vi "Get_All_Sensor_Inputs.vi"(11 "Camera Inputs":T1) -> (3 "Input_Sensors":T2)   [LabVIEW 2012]
uses:
  Inputs_All.ctl
  Flywheel/Sensor_Inputs_FlyWheel.ctl
  tankdrive/Input_Sensors_Drive.ctl
  Conveyor/Sensor_Input_Conveyor.ctl
  Conveyor/Sensor_Input_ConveyorV2.ctl
  Turret/Inputs_Sensors_Turret.ctl
  Inputs_Camera.ctl
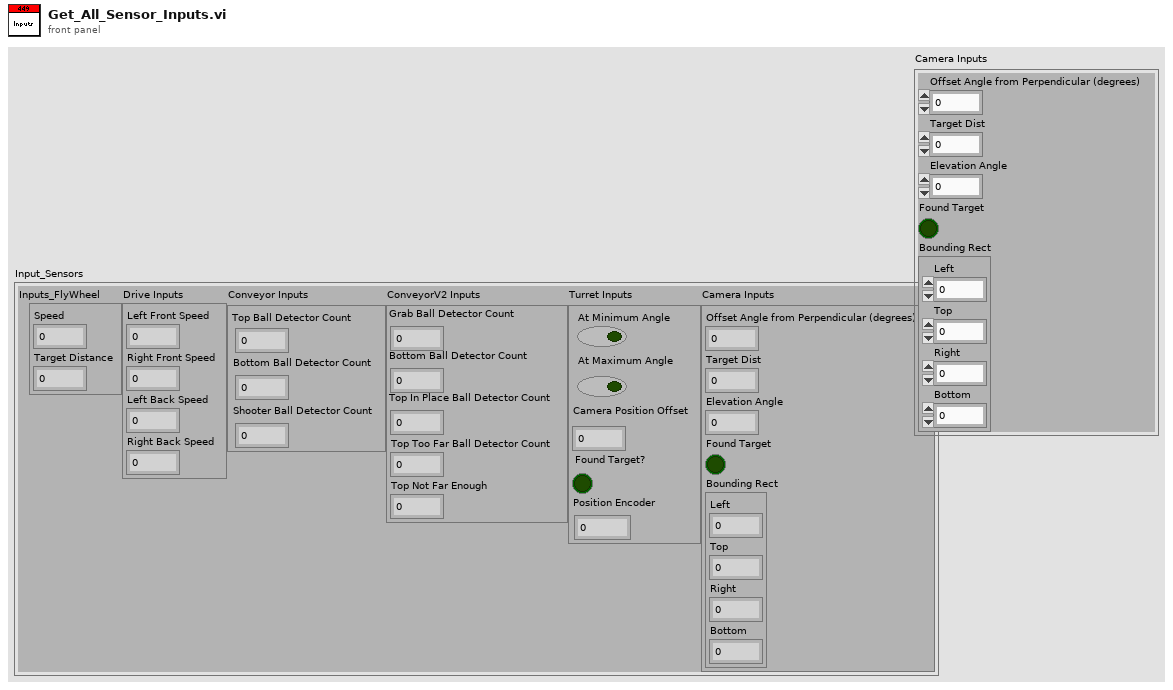
[diagram p1: front panel]
types:
  T1 = typedef "Inputs_Camera.ctl" = cluster{"Offset Angle from Perpendicular (degrees)":dbl, "Target Dist":dbl, "Elevation Angle":dbl, "Found Target":bool, "Bounding Rect":cluster{"Left":dbl, "Top":dbl, "Right":dbl, "Bottom":dbl}}
  T2 = typedef "Inputs_All.ctl" = cluster{"Inputs_FlyWheel":T3, "Drive Inputs":T4, "Conveyor Inputs":T5, "ConveyorV2 Inputs":T6, "Turret Inputs":T7, "Camera Inputs":T1}
  T3 = typedef "Sensor_Inputs_FlyWheel.ctl" = cluster{"Speed":dbl, "Target Distance":dbl}
  T4 = typedef "Input_Sensors_Drive.ctl" = cluster{"Left Front Speed":dbl, "Right Front Speed":dbl, "Left Back Speed":dbl, "Right Back Speed":dbl}
  T5 = typedef "Sensor_Input_Conveyor.ctl" = cluster{"Top Ball Detector Count":i32, "Bottom Ball Detector Count":i32, "Shooter Ball Detector Count":i32}
  T6 = typedef "Sensor_Input_ConveyorV2.ctl" = cluster{"Grab Ball Detector Count":i32, "Bottom Ball Detector Count":i32, "Top In Place Ball Detector Count":i32, "Top Too Far Ball Detector Count":i32, "Top Not Far Enough":i32}
  T7 = typedef "Inputs_Sensors_Turret.ctl" = cluster{"At Minimum Angle":bool, "At Maximum Angle":bool, "Camera Position Offset":dbl, "Found Target?":bool, "Position Encoder":dbl}
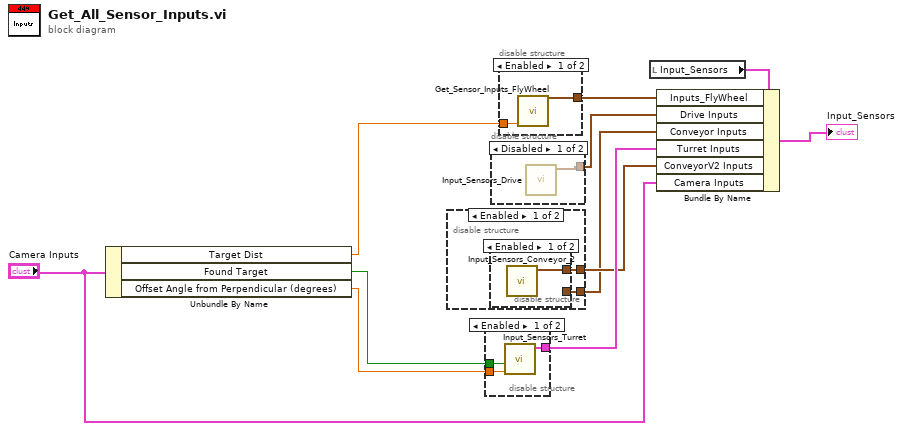
[diagram p0: block diagram]
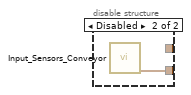
[diagram p2: hidden frame]
diagram:
  n1 = Unbundle By Name("Camera Inputs") -> ("Target Dist"=w6:dbl, "Found Target"=w4:bool, "Offset Angle from Perpendicular (degrees)"=w5:dbl)
  n2 = disable-structure shown="Enabled" {
    disable-tunnel: [w13 _] -> w3
    disable-tunnel: [w12 _] -> w2
    frame Enabled {
      n3 = disable-structure shown="Enabled" {
        disable-tunnel: [w14 _] -> w13
        disable-tunnel: [_ w15] -> w12
        frame Enabled {
          n4 = call "Input_Sensors_Conveyor_2.vi"() -> ("ConveyorV2 Inputs"=w14:T6)  [unwired: 11 in]
        }
        frame Disabled {
          n5 = call "Input_Sensors_Conveyor.vi"() -> ("Conveyor Sensor Inputs"=w15:T5)  [unwired: 10 in, 1 out]
        }
      }
    }
    frame Disabled {
    }
  }
  n6 = disable-structure shown="Enabled" {
    disable-tunnel: [w18 _] -> w7
    disable-tunnel: w5 -> [w17 _]
    disable-tunnel: w4 -> [w16 _]
    frame Enabled {
      n7 = call "Input_Sensors_Turret.vi"("Camera Hozinontal Angle Offset"=w17, "Found Target"=w16) -> ("Turret Sensor Inputs"=w18:T7)  [unwired: 9 in]
    }
    frame Disabled {
    }
  }
  n8 = disable-structure shown="Disabled" {
    disable-tunnel: [w19 _] -> w8
    frame Disabled {
      n9 = call "Input_Sensors_Drive.vi"() -> ("Drive Inputs"=w19:T4)  [unwired: 11 in]
    }
    frame Enabled {
    }
  }
  n10 = disable-structure shown="Enabled" {
    disable-tunnel: [w21 _] -> w9
    disable-tunnel: w6 -> [w20 _]
    frame Enabled {
      n11 = call "Get_Sensor_Inputs_FlyWheel.vi"("Target Dist"=w20) -> ("Sensor_Inputs_FlyWheel"=w21:T3)  [unwired: 9 in]
    }
    frame Disabled {
    }
  }
  n12 = local read "Input_Sensors"() -> (w11:T2)
  n13 = Bundle By Name(cluster=w11, "Inputs_FlyWheel"=w9, "Drive Inputs"=w8, "Conveyor Inputs"=w2, "Turret Inputs"=w7, "ConveyorV2 Inputs"=w3, "Camera Inputs"="Camera Inputs") -> (→"Input_Sensors":T2)
